vi "LJUD UE9RAW CommReset.vi"(5 "Comm Settings":T1={"Open LabJack "=TRUE, "Use USB"=TRUE, "IP Address"="192.168.1.209", "PortA"=52360, "PortB"=0}, 8 "error in (no error)":errorcluster, 11 "Handle In":i32) -> (0 "error out":errorcluster, 3 "Handle Out":i32)   [LabVIEW 2021]
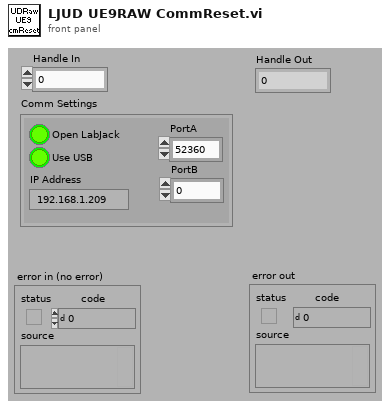
[diagram p1: front panel]
types:
  T1 = cluster{"Open LabJack ":bool, "Use USB":bool, "IP Address":string, "PortA":u16, "PortB":u16}
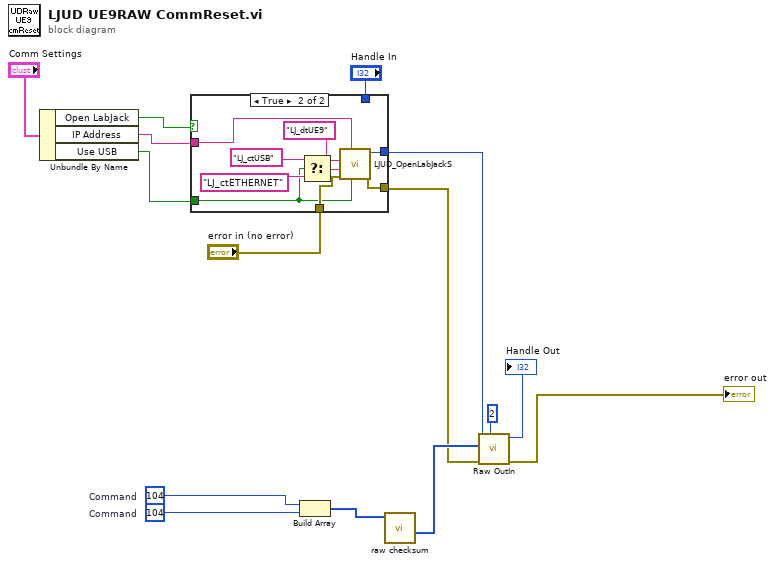
[diagram p0: block diagram]
diagram:
  w13 = u8 104  # Command
  w15 = u8 104  # Command
  n1 = Unbundle By Name("Comm Settings") -> ("Open LabJack"=w1:bool, "IP Address"=w2:string, "Use USB"=w3:bool)
  n2 = case shown="True" w1 {
    tunnel: w2 -> [_ w20]
    tunnel: "error in (no error)" -> [w17 w24]
    tunnel: [w17 w23] -> w5
    tunnel: [w16 w21] -> w6
    tunnel: w3 -> [_ w22]
    tunnel: "Handle In" -> [w16 _]
    frame False {
    }
    frame True {
      n3 = Select(t="LJ_ctUSB" ("ConnectionType"), s=w22, f="LJ_ctETHERNET" ("ConnectionType")) -> (s? t:f=w18:string)
      n4 = call "LJUD_OpenLabJackS.vi"("FirstFound"=w22, "Address"=w20, "error in"=w24, "ConnectionType"=w18, "DeviceType"="LJ_dtUE9") -> ("error out"=w23:errorcluster, "Handle"=w21:i32)  [unwired: 4 in, 1 out]
    }
  }
  n5 = Build Array(w13, w15) -> (w14:u8[])
  n6 = call "raw checksum.vi"("Array"=w14) -> ("Array Output"=w12:u8[])  [unwired: 3 in, 7 out]
  n7 = call "Raw OutIn.vi"("# of bytes to read in"=2 ("# of bytes to read"), "error in"=w5, "Raw Out"=w12, "Handle In"=w6) -> ("error out"=→"error out":errorcluster, "Handle Out"=→"Handle Out":i32)  [unwired: 4 in, 2 out]
